vi "Create Transfer Group Bundle.vi"(11 "Transfer Groups":refnum<class "Transfer Group.lvclass">[](array[class])) -> (3 "Transfer Group Bundles":refnum<class "Scheduler Transfer Group Bundle.lvclass">[](array[class]))   [LabVIEW 2017, in "DSF Core.lvlib" / "Scheduler Transfer Group Bundle.lvclass"]
uses:
  Scheduler Transfer Group Bundle.lvclass
  Transfer Group/Transfer Group.lvclass
  Transfer Group/Transfer Group.lvclass/Transfer Group.ctl
  Scheduler Transfer Group Bundle.lvclass/Scheduler Transfer Group Bundle.ctl
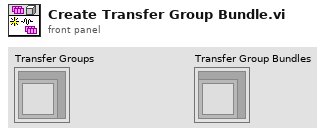
[diagram p1: front panel]
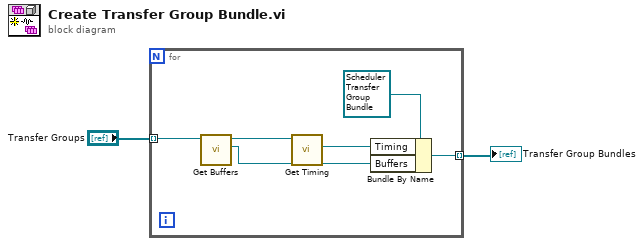
[diagram p0: block diagram]
diagram:
  n1 = for {
    tunnel: "Transfer Groups" -> [w5] mode=indexing
    tunnel: [w6] -> w1 mode=indexing
    n2 = call "Get Buffers.vi"("Transfer Group in"=w5) -> ("Buffers"=w3:refnum<class "Buffers.lvclass">, "Transfer Group out"=w4:refnum<class "Transfer Group.lvclass">)  [unwired: 9 in]
    n3 = call "Get Timing.vi"("Transfer Group in"=w4) -> ("Timing"=w7:refnum<class "Transfer Group Timing.lvclass">)  [unwired: 9 in, 1 out]
    n4 = Bundle By Name(cluster=refnum<class "Scheduler Transfer Group Bundle.lvclass"> refnum ("DSF Core.lvlib:Scheduler Transfer Group Bundle.lvclass"), "Timing"=w7, "Buffers"=w3) -> (w6:refnum<class "Scheduler Transfer Group Bundle.lvclass">)
  }
  "Transfer Group Bundles" <- w1
